vi "诊断标定3 - 副本.vi"(8 "CAN端口":u16(ring), 9 "设备索引号":u16(ring), 10 "CAN卡类型":u32(ring)=21) -> ()   [LabVIEW 2013] (continued)
                      frame Enabled {
                      }
                    }
                    n3542 = global write "读配置文件全局2.vi" "从板号判定"(w4888) -> ()
                    n3543 = global write "读配置文件全局2.vi" "通道电压判定"(w4888) -> ()
                    n3544 = global write "读配置文件全局2.vi" "保险位置判定"(w4888) -> ()
                    n3545 = global write "读配置文件全局2.vi" "二级故障判定"(w4888) -> ()
                    n3546 = global write "读配置文件全局2.vi" "三级故障判定"(w4888) -> ()
                    n3547 = global write "读配置文件全局2.vi" "一级故障判定"(w4888) -> ()
                    n3548 = global write "读配置文件全局2.vi" "电压起始值判定"(w4888) -> ()
                    n3549 = global write "读配置文件全局2.vi" "温度起始值判定"(w4888) -> ()
                  }
                }
              }
              frame #1 {
                (unwired) "均衡参数"
                # "去掉加热控制信息 20140106"
                n3550 = local read "主从选择"() -> (w4892:enum32{"主板", "从板"})
                n3551 = case shown="\"主板\", 默认" w4892 {
                  tunnel: [string[] ["项目信息", "一级故障阀值", "二级故障阀值", "三级故障阀值", "加热控制信息", "充电控制信息", "电池信息", "二维码"] string[] ["从板信息", "一级故障阀值", "二级故障阀值", "三级故障阀值", "二维码"]] -> w4891
                  frame "主板", Default {
                  }
                  frame "从板" {
                  }
                }
                n3552 = Array Size(array=w4891) -> (size(s)=w4890:i32)
                n3553 = for {
                  tunnel: w4891 -> [w4908] mode=indexing
                  tunnel: w4892 -> [w4896]
                  tunnel: w4890 -> [w4900]
                  tunnel: [w4895] -> w4889
                  i -> [w4897]
                  n3554 = case shown="\"主板\", 默认" w4896 {
                    tunnel: [w5204 w5235] -> w4902
                    tunnel: [w5203 w5236] -> w4903
                    tunnel: w4908 -> [w5200 w5232]
                    tunnel: [u8 0 ("板号") w5233] -> w4907
                    tunnel: [u8 0 ("板号") u8 0 ("板号")] -> w4906
                    tunnel: [w5199 w5231] -> w4904
                    frame "主板", Default {
                      n3555 = case shown="\"二维码\"" w5200 {
                        tunnel: [_ u8[] [1, 2, 3, 4, 5, 6, 13, 8, 7, 9, 10, 11, 12] u8[] [1] u8[] [1] u8[] [2] u8[] [3] u8[] [1] u8[] [2] u8[] [1, 2, 3] u8[] [1, 2, 3, 4]] -> w5204
                        tunnel: [_ u8 128 ("命令") u8 140 ("命令") u8 129 ("命令") u8 129 ("命令") u8 129 ("命令") u8 130 ("命令") u8 130 ("命令") u8 131 ("命令") u8 132 ("命令")] -> w5203
                        tunnel: [_ string[] ["产品编号", "电压个数", "通道电压数", "电压起始值", "温度个数", "温度起始值", "保险位置", "电池额定实际容量", "SOC", "配置文件版本", "参数修改记录", "车牌号", "SOH"] string[] ["读二维码"] string[] ["一级故障阀值"] string[] ["二级故障阀值"] string[] ["三级故障阀值"] string[] ["加热控制参数"] string[] ["充电控制参数"] _ string[] ["电池信息1", "电池包组号", "充放电安时", "电池充放电次数"]] -> w5199
                        frame "假", Default {
                        }
                        frame "项目信息" {
                        }
                        frame "二维码" {
                        }
                        frame "一级故障阀值" {
                        }
                        frame "二级故障阀值" {
                        }
                        frame "三级故障阀值" {
                        }
                        frame "加热控制信息" {
                        }
                        frame "充电控制信息" {
                        }
                        frame "历史信息" {
                        }
                        frame "电池信息" {
                        }
                      }
                    }
                    frame "从板" {
                      n3556 = case shown="\"二维码\"" w5232 {
                        tunnel: [_ u8 0 ("命令") u8 10 ("命令") u8 2 ("命令") u8 2 ("命令") u8 2 ("命令") u8 3 ("命令") u8 6 ("命令")] -> w5236
                        tunnel: [_ u8[] [6, 1, 2, 3, 4, 5] u8[] [1] u8[] [1] u8[] [2] u8[] [3] u8[] [1, 2, 3, 4, 5, 6, 7] u8[] [1, 2]] -> w5235
                        tunnel: [_ string[] ["从板号", "电压起始值", "通道电压节数", "保险位置", "温度起始值", "加热控制参数"] string[] ["读二维码"] string[] ["一级故障阀值"] string[] ["二级故障阀值"] string[] ["三级故障阀值"] string[] ["电池包信息1", "电池包序号", "充放电安时", "充电次数时间", "SOC", "车牌号", "充电参数"] string[] ["均衡阀值", "充电结束电压"]] -> w5231
                        frame "假", Default {
                        }
                        frame "从板信息" {
                        }
                        frame "二维码" {
                        }
                        frame "一级故障阀值" {
                        }
                        frame "二级故障阀值" {
                        }
                        frame "三级故障阀值" {
                        }
                        frame "快换参数" {
                        }
                        frame "均衡参数" {
                        }
                      }
                      n3557 = local read "从板号"() -> (w5233:u8)
                    }
                  }
                  n3558 = Increment(x=w4897) -> (x+1=w4899:i32)
                  n3559 = Equal?(x=w4900, y=w4899) -> (x = y?=w4898:bool)
                  n3560 = case shown="\"从板\"" w4896 {
                    tunnel: w4897 -> [w5170 w5184]
                    frame "主板", Default {
                      n3561 = case shown="0, 默认" w5170 {
                        tunnel: [T8."项目信息" ("主从板") T8."一级故障阀值" ("主从板") T8."二级故障阀值" ("主从板") T8."三级故障阀值" ("主从板") T8."控制参数" ("主从板") T8."电池信息" ("主从板")] -> w5169
                        frame 0, Default {
                          n3562 = local write "1"(TRUE ("1")) -> ()
                        }
                        frame 1 {
                          n3563 = local write "1 2"(TRUE ("1 2")) -> ()
                        }
                        frame 2 {
                          n3564 = local write "1 3"(TRUE ("1 3")) -> ()
                        }
                        frame 3 {
                          n3565 = local write "1 4"(TRUE ("1 4")) -> ()
                        }
                        frame 4, 5 {
                          n3566 = local write "1 5"(TRUE ("1 5")) -> ()
                        }
                        frame 6 {
                          n3567 = local write "1 11"(TRUE ("1 11")) -> ()
                        }
                      }
                      n3568 = local write "主板2"(w5169) -> ()
                    }
                    frame "从板" {
                      n3569 = case shown="4" w5184 {
                        tunnel: [T19."从板信息" ("等级 2") T19."从板信息" ("等级 2") T19."一级故障阀值" ("等级 2") T19."二级故障阀值" ("等级 2") T19."三级故障阀值" ("等级 2") T19."快换参数" ("等级 2") T14."从板信息" ("等级 2")] -> w5183
                        frame 99, Default {
                          n3570 = local write "1 6"(TRUE ("1 6")) -> ()
                        }
                        frame 0 {
                          n3571 = local write "1 6"(TRUE ("1 6")) -> ()
                        }
                        frame 1 {
                          n3572 = local write "1 7"(TRUE ("1 7")) -> ()
                        }
                        frame 2 {
                          n3573 = local write "1 8"(TRUE ("1 8")) -> ()
                        }
                        frame 3 {
                          n3574 = local write "1 9"(TRUE ("1 9")) -> ()
                        }
                        frame 5 {
                          n3575 = local write "1 10"(TRUE ("1 10")) -> ()
                        }
                        frame 4 {
                          n3576 = local write "1 12"(TRUE ("1 10")) -> ()
                        }
                      }
                      n3577 = local write "等级 2"(w5183) -> ()
                    }
                  }
                  n3578 = Array Size(array=w4902) -> (size(s)=w4901:i32)
                  n3579 = local write "命令"(w4903) -> ()
                  n3580 = Build Array(w4906) -> (w4905:u8[])
                  n3581 = while {
                    tunnel: w4903 -> [w4940]
                    tunnel: w4907 -> [w4939]
                    tunnel: w4905 -> [w4938]
                    tunnel: w4901 -> [w4934]
                    tunnel: w4898 -> [w4937]
                    tunnel: w4896 -> [w4931]
                    tunnel: [w4930] -> w4895
                    shift-right: [w4929] -> _
                    shift-left: w4904 -> [w4910]
                    shift-right: [w4920] -> _
                    shift-left: w4902 -> [w4909]
                    i -> [w4935]
                    stop <- w4930 stop-if-true
                    n3582 = Array Size(array=w4910) -> (size(s)=w4928:i32)
                    n3583 = local read "强制终止读写标记"() -> (w4926:bool)
                    n3584 = Increment(x=w4935) -> (x+1=w4936:i32)
                    n3585 = Greater Than 0?(x=w4928) -> (x > 0?=w4927:bool)
                    n3586 = Equal?(x=w4934, y=w4936) -> (x = y?=w4932:bool)
                    n3587 = Delete From Array(array=w4910, length=1 ("长度"), index=0 ("索引")) -> (deleted portion=w4916:string[], array with subset deleted=w4921:string[])
                    n3588 = Index Array(array=w4916, index=0 ("索引")) -> (element=w4914:string)
                    n3589 = Delete From Array(array=w4909, length=1 ("长度"), index=0 ("索引")) -> (deleted portion=w4912:u8[], array with subset deleted=w4917:u8[])
                    n3590 = Index Array(array=w4912, index=0 ("索引")) -> (element=w4911:u8)
                    n3591 = Not(x=w4926) -> (.not. x?=w4925:bool)
                    n3592 = And(x=w4925, y=w4927) -> (x .and. y?=w4924:bool)
                    n3593 = case shown="真" w4924 {
                      tunnel: w4940 -> [_ w4956]
                      tunnel: w4911 -> [_ w4955]
                      tunnel: w4939 -> [_ w4954]
                      tunnel: w4938 -> [_ w4953]
                      tunnel: w4914 -> [_ w4952]
                      tunnel: w4937 -> [_ w4951]
                      tunnel: w4932 -> [_ w4950]
                      tunnel: w4931 -> [_ w4949]
                      tunnel: [string[] [] w4945] -> w4929
                      tunnel: w4921 -> [_ w4948]
                      tunnel: [u8[] [] w4943] -> w4920
                      tunnel: w4917 -> [_ w4947]
                      tunnel: w4910 -> [_ w4946]
                      tunnel: w4909 -> [_ w4944]
                      frame False {
                      }
                      frame True {
                        n3594 = while {
                          tunnel: w4956 -> [w4972]
                          tunnel: w4955 -> [w4971]
                          tunnel: w4954 -> [w4970]
                          tunnel: w4953 -> [w4969]
                          tunnel: w4952 -> [w4967]
                          tunnel: w4951 -> [w4966]
                          tunnel: w4950 -> [w4965]
                          tunnel: w4949 -> [w4964]
                          tunnel: w4948 -> [w4960]
                          tunnel: w4947 -> [w4958]
                          tunnel: w4946 -> [w4961]
                          tunnel: [w4962] -> w4945
                          tunnel: w4944 -> [w4959]
                          tunnel: [w4957] -> w4943
                          i -> [w4963]
                          stop <- w4968 stop-if-true
                          n3595 = stacked-sequence {
                            seq-local: [_ _ _ _ w5119 _ _] -> [_ _ _ _ _ w5135 _]
                            tunnel: w4972 -> [_ _ _ w5111 _ _ _]
                            tunnel: w4971 -> [_ _ _ w5110 _ _ _]
                            tunnel: w4970 -> [_ _ _ w5109 _ _ _]
                            tunnel: w4969 -> [_ _ _ w5108 _ _ _]
                            tunnel: [_ _ _ _ w5120 _ _] -> w4968
                            tunnel: w4967 -> [w4974 _ _ _ _ w5134 _]
                            tunnel: w4966 -> [_ _ _ _ _ _ w5162]
                            tunnel: w4965 -> [_ _ _ _ _ _ w5160]
                            tunnel: w4964 -> [w4973 _ _ _ _ _ _]
                            tunnel: w4963 -> [_ _ _ _ _ _ _]
                            tunnel: [_ _ _ _ _ w5133 _] -> w4962
                            tunnel: w4961 -> [_ _ _ _ _ w5132 _]
                            tunnel: w4960 -> [_ _ _ _ _ w5131 _]
                            tunnel: w4959 -> [_ _ _ _ _ w5130 _]
                            tunnel: w4958 -> [_ _ _ _ _ w5129 _]
                            tunnel: [_ _ _ _ _ w5128 _] -> w4957
                            frame #0 {
                              n3596 = case shown="\"从板\"" w4973 {
                                tunnel: w4974 -> [w4975 w5066]
                                frame "主板", Default {
                                n3597 = case shown="\"电压个数\"" w4975 {
                                frame "假", Default {
                                }
                                frame "产品编号" {
                                n3598 = control-ref of="产品编号"() -> (w4977:refnum<vi>)
                                n3599 = property class="Str"(reference=w4977, "Value"="") -> ()  [unwired: 1 in, 2 out]
                                }
                                frame "电压个数" {
                                n3600 = local read "从板个数"() -> (w4978:dbl)
                                n3601 = control-ref of="项目信息"() -> (w4982:refnum<vi>)
                                n3602 = for {
                                N: w4978 -> [_]
                                tunnel: [""] -> w4981 mode=indexing
                                }
                                n3603 = call "表格数据输入-8.6.vi"("行数"=u32 0, "列数"=u32 1, "字符串数组"=w4981, "表格引用"=w4982) -> ()  [unwired: 8 in]
                                }
                                frame "通道电压数" {
                                n3604 = disable-structure shown="禁用" {
                                frame Disabled {
                                n3605 = control-ref of="项目信息"() -> (w4988:refnum<vi>)
                                n3606 = for {
                                N: 20 -> [_]
                                tunnel: [""] -> w4987 mode=indexing
                                }
                                n3607 = local read "从板个数"() -> (w4989:dbl)
                                n3608 = Increment(x=w4989) -> (x+1=w4985:dbl)
                                n3609 = call "表格数据输入-8.6.vi"("行数"=w4985, "列数"=u32 1, "字符串数组"=w4987, "表格引用"=w4988) -> ()  [unwired: 8 in]
                                }
                                frame Enabled {
                                }
                                }
                                }
                                frame "电压起始值" {
                                n3610 = disable-structure shown="禁用" {
                                frame Disabled {
                                n3611 = local read "从板个数"() -> (w4993:dbl)
                                n3612 = Increment(x=w4993) -> (x+1=w4992:dbl)
                                n3613 = control-ref of="项目信息"() -> (w4999:refnum<vi>)
                                n3614 = for {
                                N: w4992 -> [_]
                                tunnel: [""] -> w4998 mode=indexing
                                }
                                n3615 = Multiply(x=u8 1, y=w4993) -> (x*y=w4995:dbl)
                                n3616 = Add(x=w4995, y=u8 21) -> (x+y=w4991:dbl)
                                n3617 = call "表格数据输入-8.6.vi"("行数"=w4991, "列数"=u32 1, "字符串数组"=w4998, "表格引用"=w4999) -> ()  [unwired: 8 in]
                                }
                                frame Enabled {
                                }
                                }
                                }
                                frame "温度个数" {
                                n3618 = local read "从板个数"() -> (w5003:dbl)
                                n3619 = Increment(x=w5003) -> (x+1=w5002:dbl)
                                n3620 = control-ref of="项目信息"() -> (w5009:refnum<vi>)
                                n3621 = for {
                                N: w5002 -> [_]
                                tunnel: [""] -> w5008 mode=indexing
                                }
                                n3622 = Multiply(x=u8 2, y=w5003) -> (x*y=w5005:dbl)
                                n3623 = Add(x=w5005, y=u8 22) -> (x+y=w5001:dbl)
                                n3624 = call "表格数据输入-8.6.vi"("行数"=w5001, "列数"=u32 1, "字符串数组"=w5008, "表格引用"=w5009) -> ()  [unwired: 8 in]
                                }
                                frame "温度起始值" {
                                n3625 = disable-structure shown="禁用" {
                                frame Disabled {
                                n3626 = local read "从板个数"() -> (w5013:dbl)
                                n3627 = Increment(x=w5013) -> (x+1=w5012:dbl)
                                n3628 = control-ref of="项目信息"() -> (w5019:refnum<vi>)
                                n3629 = for {
                                N: w5012 -> [_]
                                tunnel: [""] -> w5018 mode=indexing
                                }
                                n3630 = Multiply(x=u8 3, y=w5013) -> (x*y=w5015:dbl)
                                n3631 = Add(x=w5015, y=u8 23) -> (x+y=w5011:dbl)
                                n3632 = call "表格数据输入-8.6.vi"("行数"=w5011, "列数"=u32 1, "字符串数组"=w5018, "表格引用"=w5019) -> ()  [unwired: 8 in]
                                }
                                frame Enabled {
                                }
                                }
                                }
                                frame "保险位置" {
                                n3633 = local read "从板个数"() -> (w5023:dbl)
                                n3634 = control-ref of="项目信息"() -> (w5029:refnum<vi>)
                                n3635 = for {
                                N: 10 -> [_]
                                tunnel: [""] -> w5028 mode=indexing
                                }
                                n3636 = Multiply(x=u8 4, y=w5023) -> (x*y=w5025:dbl)
                                n3637 = Add(x=w5025, y=u8 24) -> (x+y=w5022:dbl)
                                n3638 = call "表格数据输入-8.6.vi"("行数"=w5022, "列数"=u32 1, "字符串数组"=w5028, "表格引用"=w5029) -> ()  [unwired: 8 in]
                                }
                                frame "电池额定实际容量" {
                                w5031 = 0.0 ("值")
                                n3639 = control-ref of="电池实际容量(A)"() -> (w5032:refnum<vi>)
                                n3640 = control-ref of="电池额定容量(A)"() -> (w5033:refnum<vi>)
                                n3641 = property class="DigNum (严格)"(reference=w5032, "Value"=w5031) -> ()  [unwired: 1 in, 2 out]
                                n3642 = property class="DigNum (严格)"(reference=w5033, "Value"=w5031) -> ()  [unwired: 1 in, 2 out]
                                }
                                frame "SOC" {
                                n3643 = control-ref of="SOC(%)"() -> (w5034:refnum<vi>)
                                n3644 = property class="DigNum (严格)"(reference=w5034, "Value"=0.0 ("值")) -> ()  [unwired: 1 in, 2 out]
                                }
                                frame "配置文件版本" {
                                n3645 = control-ref of="配置文件版本"() -> (w5036:refnum<vi>)
                                n3646 = property class="Str"(reference=w5036, "Value"="" ("值")) -> ()  [unwired: 1 in, 2 out]
                                }
                                frame "参数修改记录" {
                                n3647 = control-ref of="使用者"() -> (w5039:refnum<vi>)
                                n3648 = control-ref of="系统时钟"() -> (w5040:refnum<vi>)
                                n3649 = property class="DigNum (严格)"(reference=w5039, "Value"=0.0 ("值")) -> ()  [unwired: 1 in, 2 out]
                                n3650 = property class="Str"(reference=w5040, "Value"="" ("值")) -> ()  [unwired: 1 in, 2 out]
                                }
                                frame "校正时钟" {
                                n3651 = control-ref of="系统时钟"() -> (w5042:refnum<vi>)
                                n3652 = property class="Str"(reference=w5042, "Value"="" ("值")) -> ()  [unwired: 1 in, 2 out]
                                }
                                frame "车牌号" {
                                n3653 = control-ref of="车架(牌)号"() -> (w5044:refnum<vi>)
                                n3654 = property class="Str"(reference=w5044, "Value"="" ("值")) -> ()  [unwired: 1 in, 2 out]
                                }
                                frame "SOH" {
                                n3655 = control-ref of="SOH(%)"() -> (w5047:refnum<vi>)
                                n3656 = property class="DigNum (严格)"(reference=w5047, "Value"=0.0 ("值")) -> ()  [unwired: 1 in, 2 out]
                                }
                                frame "一级故障阀值" {
                                n3657 = local write "一级故障"(T10 {"总电压过高"=0.0, "整组电压不均衡"=0.0, "SOC过高"=0.0, "单体电压过高"=0.0, "总电压过低"=0.0, "温度过高"=0.0, "温度过低"=0.0, "单组电压不均衡"=0.0, "整组温度不均衡"=0.0, "单组温度不均衡"=0.0, "单体电压过低"=0.0, "充电电流过高"=0.0, "放电电流过高"=0.0, "SOC过低"=0.0, "内阻过大"=0.0, "极柱温度过高"=0.0, "SOH过低"=0.0} ("一级故障")) -> ()
                                }
                                frame "二级故障阀值" {
                                n3658 = local write "一级故障 2"(T10 {"总电压过高"=0.0, "整组电压不均衡"=0.0, "SOC过高"=0.0, "单体电压过高"=0.0, "总电压过低"=0.0, "温度过高"=0.0, "温度过低"=0.0, "单组电压不均衡"=0.0, "整组温度不均衡"=0.0, "单组温度不均衡"=0.0, "单体电压过低"=0.0, "充电电流过高"=0.0, "放电电流过高"=0.0, "SOC过低"=0.0, "内阻过大"=0.0, "极柱温度过高"=0.0, "SOH过低"=0.0} ("一级故障")) -> ()
                                }
                                frame "三级故障阀值" {
                                n3659 = local write "一级故障 3"(T10 {"总电压过高"=0.0, "整组电压不均衡"=0.0, "SOC过高"=0.0, "单体电压过高"=0.0, "总电压过低"=0.0, "温度过高"=0.0, "温度过低"=0.0, "单组电压不均衡"=0.0, "整组温度不均衡"=0.0, "单组温度不均衡"=0.0, "单体电压过低"=0.0, "充电电流过高"=0.0, "放电电流过高"=0.0, "SOC过低"=0.0, "内阻过大"=0.0, "极柱温度过高"=0.0, "SOH过低"=0.0} ("一级故障")) -> ()
                                }
                                frame "加热控制参数" {
                                n3660 = local write "加热控制参数"(T11 {"风机开启温度"=0.0, "风机关闭温度"=0.0, "加热开启温度"=0.0, "加热关闭温度"=0.0, "风机开启温差"=0.0, "风机关闭温差"=0.0, "加热关闭温差"=0.0} ("加热控制参数")) -> ()
                                }
                                frame "充电控制参数" {
                                n3661 = local write "一级故障 5"(T12 {"最大允许单体电压"=0.0, "最大允许总电压"=0.0, "最小允许单体电压"=0.0, "最大允许充电电流"=0.0, "最小允许充电电流"=0.0, "最大允许充电温度"=0.0, "最小允许充电温度"=0.0, "电流步长"=0.0} ("一级故障 5")) -> ()
                                }
                                frame "电池信息1" {
                                w5053 = ""
                                w5054 = 0.0 ("电池串联")
                                n3662 = local read "电池信息"() -> (w5056:T13)
                                n3663 = Bundle By Name(cluster=w5056, "电池串联"=w5054, "电池并联"=w5054, "电池包额定容量"=w5054, "电池包额定能量(kWh)"=w5054, "电池包额定总电压"=w5054, "实际容量"=w5054, "电池厂家"=w5053, "电池类型"=w5053, "电池生产日期"=w5053) -> (w5055:T13)
                                n3664 = local write "电池信息"(w5055) -> ()
                                }
                                frame "电池包组号" {
                                n3665 = local read "电池信息"() -> (w5059:T13)
                                n3666 = Bundle By Name(cluster=w5059, "电池包组号"="") -> (w5058:T13)
                                n3667 = local write "电池信息"(w5058) -> ()
                                }
                                frame "充放电安时" {
                                w5060 = 0.0 ("累计充电总安时")
                                n3668 = local read "电池信息"() -> (w5062:T13)
                                n3669 = Bundle By Name(cluster=w5062, "累计充电总安时"=w5060, "累计放电总安时"=w5060) -> (w5061:T13)
                                n3670 = local write "电池信息"(w5061) -> ()
                                }
                                frame "电池充放电次数" {
                                w5063 = 0.0 ("累计充电总安时")
                                n3671 = local read "电池信息"() -> (w5065:T13)
                                n3672 = Bundle By Name(cluster=w5065, "电池充满次数"=w5063, "电池放空次数"=w5063, "电池充电次数"=w5063) -> (w5064:T13)
                                n3673 = local write "电池信息"(w5064) -> ()
                                }
                                }
                                }
                                frame "从板" {
                                n3674 = case shown="\"电压起始值\"" w5066 {
                                frame "假", Default {
                                }
                                frame "电压起始值" {
                                n3675 = control-ref of="项目信息 2"() -> (w5067:refnum<vi>)
                                n3676 = for {
                                N: 1 -> [_]
                                tunnel: [""] -> w5071 mode=indexing
                                }
                                n3677 = call "表格数据输入-8.6.vi"("行数"=u32 0, "列数"=u32 1, "字符串数组"=w5071, "表格引用"=w5067) -> ()  [unwired: 8 in]
                                }
                                frame "通道电压个数" {
                                n3678 = control-ref of="项目信息 2"() -> (w5073:refnum<vi>)
                                n3679 = for {
                                N: 5 -> [_]
                                tunnel: [""] -> w5077 mode=indexing
                                }
                                n3680 = call "表格数据输入-8.6.vi"("行数"=u32 22, "列数"=u32 1, "字符串数组"=w5077, "表格引用"=w5073) -> ()  [unwired: 8 in]
                                }
                                frame "保险位置" {
                                n3681 = control-ref of="项目信息 2"() -> (w5079:refnum<vi>)
                                n3682 = for {
                                N: 10 -> [_]
                                tunnel: [""] -> w5083 mode=indexing
                                }
                                n3683 = call "表格数据输入-8.6.vi"("行数"=u32 2, "列数"=u32 1, "字符串数组"=w5083, "表格引用"=w5079) -> ()  [unwired: 8 in]
                                }
                                frame "温度起始值" {
                                n3684 = control-ref of="项目信息 2"() -> (w5085:refnum<vi>)
                                n3685 = for {
                                N: 1 -> [_]
                                tunnel: [""] -> w5089 mode=indexing
                                }
                                n3686 = call "表格数据输入-8.6.vi"("行数"=u32 1, "列数"=u32 1, "字符串数组"=w5089, "表格引用"=w5085) -> ()  [unwired: 8 in]
                                }
                                frame "加热控制参数" {
                                n3687 = local write "加热控制参数"(T11 {"风机开启温度"=0.0, "风机关闭温度"=0.0, "加热开启温度"=0.0, "加热关闭温度"=0.0, "风机开启温差"=0.0, "风机关闭温差"=0.0, "加热关闭温差"=0.0} ("加热控制参数")) -> ()
                                }
                                frame "一级故障阀值" {
                                n3688 = local write "一级故障 6"(T15 {"电压过高"=0.0, "电压过低"=0.0, "温度过高"=0.0, "温度过低"=0.0, "电压不均衡(V)"=0.0, "温度不均衡"=0.0, "SOC过低"=0.0} ("一级故障 6")) -> ()
                                }
                                frame "二级故障阀值" {
                                n3689 = local write "一级故障 7"(T15 {"电压过高"=0.0, "电压过低"=0.0, "温度过高"=0.0, "温度过低"=0.0, "电压不均衡(V)"=0.0, "温度不均衡"=0.0, "SOC过低"=0.0} ("一级故障 7")) -> ()
                                }
                                frame "三级故障阀值" {
                                n3690 = local write "一级故障 8"(T15 {"电压过高"=0.0, "电压过低"=0.0, "温度过高"=0.0, "温度过低"=0.0, "电压不均衡(V)"=0.0, "温度不均衡"=0.0, "SOC过低"=0.0} ("一级故障 7")) -> ()
                                }
                                frame "均衡参数" {
                                n3691 = local write "均衡参数"(T17 {"充电结束电压(90%)"=0.0, "充电结束电压(91%)"=0.0, "充电结束电压(92%)"=0.0, "充电结束电压(93%)"=0.0, "充电结束电压(94%)"=0.0, "均衡计算-电压高阀值1级"=0.0, "均衡计算-电压高阀值2级"=0.0, "均衡计算-电压低阀值1级"=0.0, "均衡计算-电压低阀值2级"=0.0, "均衡计算-最低电压阀值"=0.0, "均衡停止-最低电压阀值"=0.0, "均衡计算-电压极差阀值"=0.0, "充电结束电压(95%)"=0.0, "充电结束电压(96%)"=0.0, "充电结束电压(97%)"=0.0, "充电结束电压(98%)"=0.0, "充电结束电压(99%)"=0.0, "充电结束电压(100%)"=0.0} ("均衡参数")) -> ()
                                }
                                frame "均衡阀值" {
                                w5096 = sgl 0.0 ("均衡计算-电压高阀值1级")
                                n3692 = local read "均衡参数"() -> (w5097:T17)
                                n3693 = Bundle By Name(cluster=w5097, "均衡计算-电压高阀值1级"=w5096, "均衡计算-电压高阀值2级"=w5096, "均衡计算-电压低阀值1级"=w5096, "均衡计算-电压低阀值2级"=w5096, "均衡计算-最低电压阀值"=w5096, "均衡停止-最低电压阀值"=w5096, "均衡计算-电压极差阀值"=w5096) -> (w5098:T17)
                                n3694 = local write "均衡参数"(w5098) -> ()
                                }
                                frame "充电结束电压" {
                                w5099 = sgl 0.0 ("均衡计算-电压高阀值1级")
                                n3695 = local read "均衡参数"() -> (w5100:T17)
                                n3696 = Bundle By Name(cluster=w5100, "充电结束电压(90%)"=w5099, "充电结束电压(91%)"=w5099, "充电结束电压(92%)"=w5099, "充电结束电压(93%)"=w5099, "充电结束电压(94%)"=w5099, "充电结束电压(95%)"=w5099, "充电结束电压(96%)"=w5099, "充电结束电压(97%)"=w5099, "充电结束电压(98%)"=w5099, "充电结束电压(99%)"=w5099, "充电结束电压(100%)"=w5099) -> (w5101:T17)
                                n3697 = local write "均衡参数"(w5101) -> ()
                                }
                                }
                                }
                              }
                            }
                            frame #1 {
                              w5102 = FALSE ("流控帧")
                              w5103 = TRUE ("流控帧 2")
                              n3698 = global write "EV05全局变量1.vi" "写入超时"(w5102) -> ()
                              n3699 = global write "EV05全局变量1.vi" "流控帧"(w5102) -> ()
                              n3700 = local write "写?"(w5102) -> ()
                              n3701 = local write "消除"(w5103) -> ()
                              n3702 = local write "控制1"(w5103) -> ()
                              n3703 = global write "EV05全局变量1.vi" "流控帧 2"(w5103) -> ()
                            }
                            frame #2 {
                              n3704 = Wait Until Next ms Multiple(millisecond multiple=u32 300 ("毫秒倍数")) -> ()  [unwired: 1 out]
                            }
                            frame #3 {
                              n3705 = local read "设备索引号"() -> (w5106:u16)
                              n3706 = local read "CAN卡类型"() -> (w5107:u32)
                              n3707 = local read "CAN端口"() -> (w5105:u16)
                              n3708 = local write "命令序号"(w5110) -> ()
                              n3709 = stacked-sequence {
                                tunnel: w5111 -> [_ w5118]
                                tunnel: w5110 -> [_ w5117]
                                tunnel: w5109 -> [_ w5116]
                                tunnel: w5108 -> [_ w5115]
                                tunnel: w5107 -> [_ w5114]
                                tunnel: w5106 -> [_ w5113]
                                tunnel: w5105 -> [_ w5112]
                                frame #0 {
                                }
                                frame #1 {
                                n3710 = call "多帧发送机制(EV05).vi"("can卡类型"=w5114, "设备索引号"=w5113, "CAN端口"=w5112, "命令"=w5118, "板号"=w5116, "命令序号"=w5117, "输入数据"=w5115) -> ()  [unwired: 1 in, 12 out]
                                }
                              }
                            }
                            frame #4 {
                              n3711 = while {
                                tunnel: [w5123] -> w5120
                                tunnel: [w5122] -> w5119
                                i -> [w5126]
                                stop <- w5123 stop-if-true
                                n3712 = local read "强制终止读写标记"() -> (w5121:bool)
                                n3713 = global read "EV05全局变量1.vi" "写入超时"() -> (w5122:bool)
                                n3714 = Greater Or Equal?(x=w5126, y=20) -> (x >= y?=w5124:bool)
                                n3715 = Compound Arithmetic op=OR(w5121, w5122, w5124) -> (w5123:bool)
                                n3716 = Wait Until Next ms Multiple(millisecond multiple=u32 100 ("毫秒倍数")) -> ()  [unwired: 1 out]
                              }
                            }
                            frame #5 {
                              n3717 = case shown="假" w5135 {
                                tunnel: w5134 -> [w5146 _]
                                tunnel: [w5141 w5158] -> w5133
                                tunnel: w5132 -> [w5140 _]
                                tunnel: w5131 -> [w5139 w5158]
                                tunnel: [w5138 w5157] -> w5128
                                tunnel: w5130 -> [w5137 _]
                                tunnel: w5129 -> [w5136 w5157]
                                frame False {
                                n3718 = local read "重试次数"() -> (w5145:u8)
                                n3719 = Increment(x=w5145) -> (x+1=w5144:u8)
                                n3720 = local write "重试次数"(w5144) -> ()
                                n3721 = Greater Or Equal?(x=w5144, y=u8 4) -> (x >= y?=w5143:bool)
                                n3722 = case shown="真" w5143 {
                                tunnel: w5146 -> [_ w5151]
                                tunnel: [w5148 w5150] -> w5141
                                tunnel: w5140 -> [w5148 _]
                                tunnel: w5139 -> [_ w5150]
                                tunnel: [w5147 w5149] -> w5138
                                tunnel: w5137 -> [w5147 _]
                                tunnel: w5136 -> [_ w5149]
                                frame False {
                                }
                                frame True {
                                n3723 = control-ref of="结果"() -> (w5153:refnum<vi>)
                                n3724 = Concatenate Strings(w5151, "     读取失败" ("字符串")) -> (w5155:string)
                                n3725 = Build Array(w5155) -> (w5152:string[])
                                n3726 = call "表格编辑.vi"("新元素/子数组"=w5152, "活动单元格:单元格背景色"=u32 16740749, "MCListbox引用句柄"=w5153) -> ()  [unwired: 9 out]
                                }
                                }
                                }
                                frame True {
                                }
                              }
                            }
                            frame #6 {
                              n3727 = And(x=w5160, y=w5162) -> (x .and. y?=w5161:bool)
                              n3728 = case shown="真" w5161 {
                                frame False {
                                }
                                frame True {
                                n3729 = local write "强制终止读写标记"(FALSE ("强制停止")) -> ()
                                n3730 = control-ref of="结果"() -> (w5165:refnum<vi>)
                                n3731 = Concatenate Strings("读取完成" ("字符串")) -> (w5167:string)
                                n3732 = Build Array(w5167) -> (w5164:string[])
                                n3733 = call "表格编辑.vi"("新元素/子数组"=w5164, "活动单元格:单元格背景色"=u32 21937, "MCListbox引用句柄"=w5165) -> ()  [unwired: 9 out]
                                }
                              }
                              n3734 = Wait (ms)(milliseconds to wait=u32 50 ("等待时间（毫秒）")) -> ()  [unwired: 1 out]
                            }
                          }
                        }
                      }
                    }
                    n3735 = local read "强制终止读写标记"() -> (w4933:bool)
                    n3736 = Or(x=w4933, y=w4932) -> (x .or. y?=w4930:bool)
                  }
                }
              }
              frame #2 {
                n3737 = case shown="假" w5258 {
                  tunnel: w5259 -> [w5260 _]
                  frame False {
                    n3738 = case shown="\"主板\", 默认" w5260 {
                      frame "主板", Default {
                        n3739 = global read "读配置文件全局.vi" "电池额定实际容量判定"() -> (w5274:bool)
                        n3740 = global read "读配置文件全局.vi" "电池充放电次数判定"() -> (w5263:bool)
                        n3741 = global read "读配置文件全局.vi" "加热控制参数判定"() -> (w5261:bool)
                        n3742 = global read "读配置文件全局.vi" "配置文件版本判定"() -> (w5273:bool)
                        n3743 = global read "读配置文件全局.vi" "充电控制参数判定"() -> (w5267:bool)
                        n3744 = global read "读配置文件全局.vi" "通道电压数判定"() -> (w5279:bool)
                        n3745 = global read "读配置文件全局.vi" "电压起始值判定"() -> (w5278:bool)
                        n3746 = global read "读配置文件全局.vi" "温度起始值判定"() -> (w5276:bool)
                        n3747 = global read "读配置文件全局.vi" "充放电安时判定"() -> (w5265:bool)
                        n3748 = global read "读配置文件全局.vi" "电池包组号判定"() -> (w5264:bool)
                        n3749 = global read "读配置文件全局.vi" "电池信息1判定"() -> (w5266:bool)
                        n3750 = global read "读配置文件全局.vi" "从板个数判定"() -> (w5282:bool)
                        n3751 = global read "读配置文件全局.vi" "产品编号判定"() -> (w5281:bool)
                        n3752 = global read "读配置文件全局.vi" "电压个数判定"() -> (w5280:bool)
                        n3753 = global read "读配置文件全局.vi" "温度个数判定"() -> (w5277:bool)
                        n3754 = global read "读配置文件全局.vi" "保险位置判定"() -> (w5275:bool)
                        n3755 = global read "读配置文件全局.vi" "一级故障判定"() -> (w5270:bool)
                        n3756 = global read "读配置文件全局.vi" "二级故障判定"() -> (w5269:bool)
                        n3757 = global read "读配置文件全局.vi" "三级故障判定"() -> (w5268:bool)
                        n3758 = global read "读配置文件全局.vi" "车牌号判定"() -> (w5272:bool)
                        n3759 = global read "读配置文件全局.vi" "SOH判定"() -> (w5271:bool)
                        n3760 = Build Array(w5282, w5281, w5280, w5279, w5278, w5277, w5276, w5275, w5274, w5273, w5272, w5271, w5270, w5269, w5268, w5267, w5266, w5265, w5264, w5263, w5261) -> (w5262:bool[])
                        n3761 = And Array Elements(Boolean array=w5262) -> (logical AND=w5283:bool)
                        n3762 = disable-structure shown="禁用" {
                          frame Disabled {
                            n3763 = global read "读配置文件全局.vi" "SOC判定"() -> ()  [unwired: 1 out]
                          }
                          frame Enabled {
                          }
                        }
                        n3764 = case shown="假" w5283 {
                          tunnel: w5262 -> [_ w5288]
                          frame True {
                            n3765 = control-ref of="结果"() -> (w5286:refnum<vi>)
                            n3766 = Build Array("全部判定成功!!!!!!!!") -> (w5287:string[])
                            n3767 = call "表格编辑.vi"("新元素/子数组"=w5287, "活动单元格:单元格背景色"=u32 6618880, "MCListbox引用句柄"=w5286) -> ()  [unwired: 9 out]
                          }
                          frame False {
                            n3768 = stacked-sequence {
                              tunnel: w5288 -> [_ w5293]
                              frame #0 {
                                n3769 = control-ref of="结果"() -> (w5291:refnum<vi>)
                                n3770 = Build Array("全部判定失败!!!!!") -> (w5292:string[])
                                n3771 = call "表格编辑.vi"("新元素/子数组"=w5292, "活动单元格:单元格背景色"=u32 16711680, "MCListbox引用句柄"=w5291) -> ()  [unwired: 9 out]
                              }
                              frame #1 {
                                n3772 = for {
                                tunnel: w5293 -> [w5295] mode=indexing
                                i -> [w5294]
                                n3773 = case shown="20" w5294 {
                                tunnel: w5295 -> [w5296 w5301 w5306 w5311 w5316 w5321 w5326 w5331 w5336 w5341 w5346 w5351 w5356 w5361 w5366 w5371 w5376 w5381 w5386 w5391 w5396 _]
                                frame 0 {
                                n3774 = case shown="假" w5296 {
                                frame False {
                                n3775 = control-ref of="结果"() -> (w5299:refnum<vi>)
                                n3776 = Build Array("从板个数判定失败!") -> (w5300:string[])
                                n3777 = call "表格编辑.vi"("新元素/子数组"=w5300, "活动单元格:单元格背景色"=u32 16711680, "MCListbox引用句柄"=w5299) -> ()  [unwired: 9 out]
                                }
                                frame True {
                                }
                                }
                                }
                                frame 1 {
                                n3778 = case shown="假" w5301 {
                                frame False {
                                n3779 = control-ref of="结果"() -> (w5304:refnum<vi>)
                                n3780 = Build Array("产品编号判定失败!") -> (w5305:string[])
                                n3781 = call "表格编辑.vi"("新元素/子数组"=w5305, "活动单元格:单元格背景色"=u32 16711680, "MCListbox引用句柄"=w5304) -> ()  [unwired: 9 out]
                                }
                                frame True {
                                }
                                }
                                }
                                frame 2 {
                                n3782 = case shown="假" w5306 {
                                frame False {
                                n3783 = control-ref of="结果"() -> (w5309:refnum<vi>)
                                n3784 = Build Array("电压个数判定失败!") -> (w5310:string[])
                                n3785 = call "表格编辑.vi"("新元素/子数组"=w5310, "活动单元格:单元格背景色"=u32 16711680, "MCListbox引用句柄"=w5309) -> ()  [unwired: 9 out]
                                }
                                frame True {
                                }
                                }
                                }
                                frame 3 {
                                n3786 = case shown="假" w5311 {
                                frame False {
                                n3787 = control-ref of="结果"() -> (w5314:refnum<vi>)
                                n3788 = Build Array("通道电压数判定失败!") -> (w5315:string[])
                                n3789 = call "表格编辑.vi"("新元素/子数组"=w5315, "活动单元格:单元格背景色"=u32 16711680, "MCListbox引用句柄"=w5314) -> ()  [unwired: 9 out]
                                }
                                frame True {
                                }
                                }
                                }
                                frame 4 {
                                n3790 = case shown="假" w5316 {
                                frame False {
                                n3791 = control-ref of="结果"() -> (w5319:refnum<vi>)
                                n3792 = Build Array("电压起始值判定失败!") -> (w5320:string[])
                                n3793 = call "表格编辑.vi"("新元素/子数组"=w5320, "活动单元格:单元格背景色"=u32 16711680, "MCListbox引用句柄"=w5319) -> ()  [unwired: 9 out]
                                }
                                frame True {
                                }
                                }
                                }
                                frame 5 {
                                n3794 = case shown="假" w5321 {
                                frame False {
                                n3795 = control-ref of="结果"() -> (w5324:refnum<vi>)
                                n3796 = Build Array("温度个数判定失败!") -> (w5325:string[])
                                n3797 = call "表格编辑.vi"("新元素/子数组"=w5325, "活动单元格:单元格背景色"=u32 16711680, "MCListbox引用句柄"=w5324) -> ()  [unwired: 9 out]
                                }
                                frame True {
                                }
                                }
                                }
                                frame 6 {
                                n3798 = case shown="假" w5326 {
                                frame False {
                                n3799 = control-ref of="结果"() -> (w5329:refnum<vi>)
                                n3800 = Build Array("温度起始值判定失败!") -> (w5330:string[])
                                n3801 = call "表格编辑.vi"("新元素/子数组"=w5330, "活动单元格:单元格背景色"=u32 16711680, "MCListbox引用句柄"=w5329) -> ()  [unwired: 9 out]
                                }
                                frame True {
                                }
                                }
                                }
                                frame 7 {
                                n3802 = case shown="假" w5331 {
                                frame False {
                                n3803 = control-ref of="结果"() -> (w5334:refnum<vi>)
                                n3804 = Build Array("保险位置判定失败!") -> (w5335:string[])
                                n3805 = call "表格编辑.vi"("新元素/子数组"=w5335, "活动单元格:单元格背景色"=u32 16711680, "MCListbox引用句柄"=w5334) -> ()  [unwired: 9 out]
                                }
                                frame True {
                                }
                                }
                                }
                                frame 8 {
                                n3806 = case shown="假" w5336 {
                                frame False {
                                n3807 = control-ref of="结果"() -> (w5339:refnum<vi>)
                                n3808 = Build Array("电池额定实际容量判定失败!") -> (w5340:string[])
                                n3809 = call "表格编辑.vi"("新元素/子数组"=w5340, "活动单元格:单元格背景色"=u32 16711680, "MCListbox引用句柄"=w5339) -> ()  [unwired: 9 out]
                                }
                                frame True {
                                }
                                }
                                }
                                frame 9 {
                                n3810 = case shown="假" w5341 {
                                frame False {
                                n3811 = control-ref of="结果"() -> (w5344:refnum<vi>)
                                n3812 = Build Array("配置文件版本判定失败!") -> (w5345:string[])
                                n3813 = call "表格编辑.vi"("新元素/子数组"=w5345, "活动单元格:单元格背景色"=u32 16711680, "MCListbox引用句柄"=w5344) -> ()  [unwired: 9 out]
                                }
                                frame True {
                                }
                                }
                                }
                                frame 10 {
                                n3814 = case shown="假" w5346 {
                                frame False {
                                n3815 = control-ref of="结果"() -> (w5349:refnum<vi>)
                                n3816 = Build Array("车牌号判定失败!") -> (w5350:string[])
                                n3817 = call "表格编辑.vi"("新元素/子数组"=w5350, "活动单元格:单元格背景色"=u32 16711680, "MCListbox引用句柄"=w5349) -> ()  [unwired: 9 out]
                                }
                                frame True {
                                }
                                }
                                }
                                frame 11 {
                                n3818 = case shown="假" w5351 {
                                frame False {
                                n3819 = control-ref of="结果"() -> (w5354:refnum<vi>)
                                n3820 = Build Array("SOH判定失败!") -> (w5355:string[])
                                n3821 = call "表格编辑.vi"("新元素/子数组"=w5355, "活动单元格:单元格背景色"=u32 16711680, "MCListbox引用句柄"=w5354) -> ()  [unwired: 9 out]
                                }
                                frame True {
                                }
                                }
                                }
                                frame 12 {
                                n3822 = case shown="假" w5356 {
                                frame False {
                                n3823 = control-ref of="结果"() -> (w5359:refnum<vi>)
                                n3824 = Build Array("一级故障阀值判定失败!") -> (w5360:string[])
                                n3825 = call "表格编辑.vi"("新元素/子数组"=w5360, "活动单元格:单元格背景色"=u32 16711680, "MCListbox引用句柄"=w5359) -> ()  [unwired: 9 out]
                                }
                                frame True {
                                }
                                }
                                }
                                frame 13 {
                                n3826 = case shown="假" w5361 {
                                frame False {
                                n3827 = control-ref of="结果"() -> (w5364:refnum<vi>)
                                n3828 = Build Array("二级故障阀值判定失败!") -> (w5365:string[])
                                n3829 = call "表格编辑.vi"("新元素/子数组"=w5365, "活动单元格:单元格背景色"=u32 16711680, "MCListbox引用句柄"=w5364) -> ()  [unwired: 9 out]
                                }
                                frame True {
                                }
                                }
                                }
                                frame 14 {
                                n3830 = case shown="假" w5366 {
                                frame False {
                                n3831 = control-ref of="结果"() -> (w5369:refnum<vi>)
                                n3832 = Build Array("三级故障阀值判定失败!") -> (w5370:string[])
                                n3833 = call "表格编辑.vi"("新元素/子数组"=w5370, "活动单元格:单元格背景色"=u32 16711680, "MCListbox引用句柄"=w5369) -> ()  [unwired: 9 out]
                                }
                                frame True {
                                }
                                }
                                }
                                frame 15 {
                                n3834 = case shown="假" w5371 {
                                frame False {
                                n3835 = control-ref of="结果"() -> (w5374:refnum<vi>)
                                n3836 = Build Array("充电控制参数判定失败!") -> (w5375:string[])
                                n3837 = call "表格编辑.vi"("新元素/子数组"=w5375, "活动单元格:单元格背景色"=u32 16711680, "MCListbox引用句柄"=w5374) -> ()  [unwired: 9 out]
                                }
                                frame True {
                                }
                                }
                                }
                                frame 16 {
                                n3838 = case shown="假" w5376 {
                                frame False {
                                n3839 = control-ref of="结果"() -> (w5379:refnum<vi>)
                                n3840 = Build Array("电池信息1判定失败!") -> (w5380:string[])
                                n3841 = call "表格编辑.vi"("新元素/子数组"=w5380, "活动单元格:单元格背景色"=u32 16711680, "MCListbox引用句柄"=w5379) -> ()  [unwired: 9 out]
                                }
                                frame True {
                                }
                                }
                                }
                                frame 17 {
                                n3842 = case shown="假" w5381 {
                                frame False {
                                n3843 = control-ref of="结果"() -> (w5384:refnum<vi>)
                                n3844 = Build Array("充放电安时判定失败!") -> (w5385:string[])
                                n3845 = call "表格编辑.vi"("新元素/子数组"=w5385, "活动单元格:单元格背景色"=u32 16711680, "MCListbox引用句柄"=w5384) -> ()  [unwired: 9 out]
                                }
                                frame True {
                                }
                                }
                                }
                                frame 18 {
                                n3846 = case shown="假" w5386 {
                                frame False {
                                n3847 = control-ref of="结果"() -> (w5389:refnum<vi>)
                                n3848 = Build Array("电池包组号判定失败!") -> (w5390:string[])
                                n3849 = call "表格编辑.vi"("新元素/子数组"=w5390, "活动单元格:单元格背景色"=u32 16711680, "MCListbox引用句柄"=w5389) -> ()  [unwired: 9 out]
                                }
                                frame True {
                                }
                                }
                                }
                                frame 19 {
                                n3850 = case shown="假" w5391 {
                                frame False {
                                n3851 = control-ref of="结果"() -> (w5394:refnum<vi>)
                                n3852 = Build Array("电池充放电次数判定失败!") -> (w5395:string[])
                                n3853 = call "表格编辑.vi"("新元素/子数组"=w5395, "活动单元格:单元格背景色"=u32 16711680, "MCListbox引用句柄"=w5394) -> ()  [unwired: 9 out]
                                }
                                frame True {
                                }
                                }
                                }
                                frame 20 {
                                n3854 = case shown="假" w5396 {
                                frame False {
                                n3855 = control-ref of="结果"() -> (w5399:refnum<vi>)
                                n3856 = Build Array("加热控制参数判定失败!") -> (w5400:string[])
                                n3857 = call "表格编辑.vi"("新元素/子数组"=w5400, "活动单元格:单元格背景色"=u32 16711680, "MCListbox引用句柄"=w5399) -> ()  [unwired: 9 out]
                                }
                                frame True {
                                }
                                }
                                }
                                frame 99, Default {
                                }
                                }
                                }
                              }
                            }
                          }
                        }
                      }
                      frame "从板" {
                        n3858 = global read "读配置文件全局2.vi" "电压起始值判定"() -> (w5409:bool)
                        n3859 = global read "读配置文件全局2.vi" "温度起始值判定"() -> (w5406:bool)
                        n3860 = global read "读配置文件全局2.vi" "加热控制参数判定"() -> (w5401:bool)
                        n3861 = global read "读配置文件全局2.vi" "通道电压判定"() -> (w5408:bool)
                        n3862 = global read "读配置文件全局2.vi" "保险位置判定"() -> (w5407:bool)
                        n3863 = global read "读配置文件全局2.vi" "一级故障判定"() -> (w5404:bool)
                        n3864 = global read "读配置文件全局2.vi" "二级故障判定"() -> (w5403:bool)
                        n3865 = global read "读配置文件全局2.vi" "三级故障判定"() -> (w5402:bool)
